vi "Init_Adapter_TCP.vi"(8 "error in (no error)":errorcluster, 11 "Siemens Ctr in":T1) -> (0 "error out":errorcluster, 3 "Siemens Ctr out":T1)   [LabVIEW 2014, in "Simatic S7.lvlib"]
uses:
  Simatic S7.lvlib
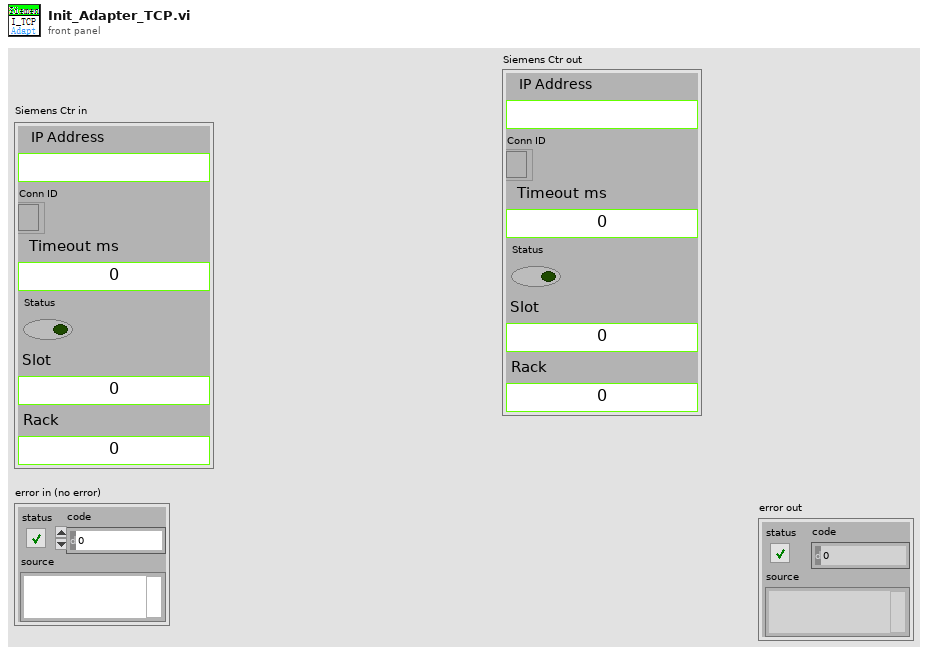
[diagram p1: front panel]
types:
  T1 = typedef "Simatic S7.lvlib/Siemens Ref.ctl" = cluster{"IP Address ":string, "Conn ID":refnum<k5>, "Timeout ms":i32, "Status":bool, "Slot":u16, "Rack":u16}
  T2 = enum16{"Standard", "Buffered", "CRLF", "Immediate"}
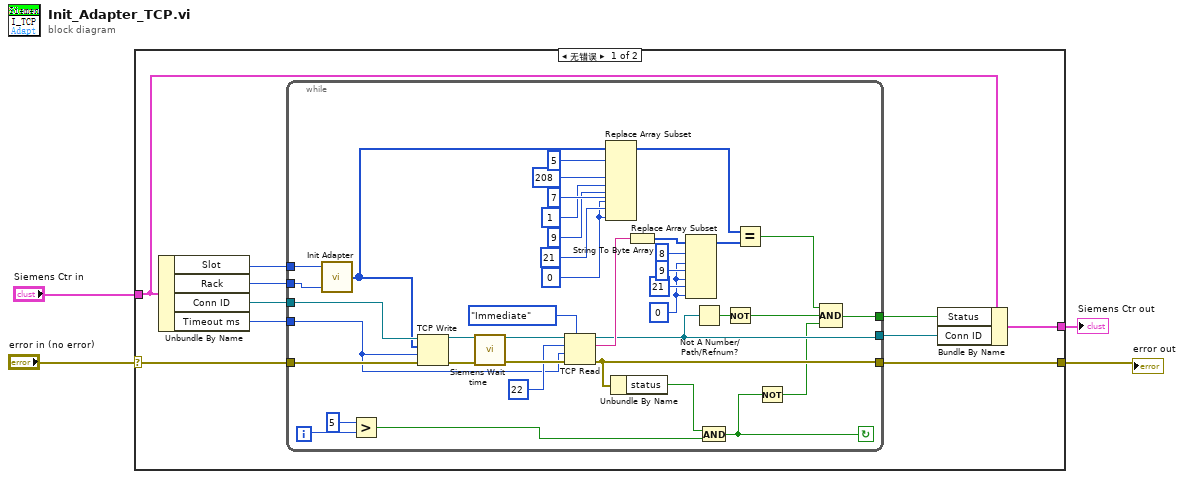
[diagram p0: block diagram]
diagram:
  n1 = case shown="无错误" "error in (no error)" {
    selector: "error in (no error)" -> [w14 w54]
    tunnel: "Siemens Ctr in" -> [w8 w53]
    tunnel: [w9 w54] -> w2
    tunnel: [w5 w53] -> w1
    frame No Error {
      n2 = Unbundle By Name(w8) -> ("Slot"=w13:u16, "Rack"=w12:u16, "Conn ID"=w11:refnum<k5>, "Timeout ms"=w10:i32)
      n3 = while {
        tunnel: w14 -> [w50]
        tunnel: w13 -> [w52]
        tunnel: w12 -> [w51]
        tunnel: w11 -> [w49]
        tunnel: w10 -> [w44]
        tunnel: [w24] -> w9
        tunnel: [w23] -> w7
        tunnel: [w15] -> w6
        i -> [w28]
        stop <- w17 continue-if-true
        w31 = u8 0 ("new element/subarray")
        w36 = u8 0 ("新元素/子数组")
        n4 = call "Init Adapter.vi"("Rack"=w51, "Slot"=w52) -> ("ISO_CR"=w35:u8[])  [unwired: 3 in]
        n5 = Greater?(x=5, y=w28) -> (0:w25:bool)
        n6 = TCP Write(connection ID=w49, data in=w35, error in (no error)=w50, 9:w44) -> (connection ID out=w46:refnum<k5>, error out=w48:errorcluster)  [unwired: 1 out]
        n7 = call "Siemens Wait time.vi"("error in (no error)"=w48) -> ("error out"=w47:errorcluster)  [unwired: 9 in, 1 out]
        n8 = TCP Read(connection ID=w46, bytes to read=22, error in (no error)=w47, 7:T2."Immediate" ("mode (standard)"), 9:w44) -> (connection ID out=w23:refnum<k5>, data out=w30:string, error out=w24:errorcluster)
        n9 = Replace Array Subset(array=w35, new element #1=u8 208 ("新元素/子数组"), index #1=5 ("索引"), new element #2=u8 1 ("新元素/子数组"), index #2=7 ("索引"), new element #3=w36, index #3=9 ("索引"), new element #4=w36, index #4=21 ("索引")) -> (w20:u8[])
        n10 = Unbundle By Name(w24) -> ("status"=w26:bool)
        n11 = String To Byte Array(string=w30) -> (unsigned byte array=w29:u8[])
        n12 = Replace Array Subset(array=w29, new element #1=w31, index #1=8 ("index"), new element #2=w31, index #2=9 ("index"), new element #3=w31, index #3=21 ("index")) -> (w21:u8[])
        n13 = Not A Number/Path/Refnum?(number/path/refnum=w23) -> (NaN/Path/Refnum?=w22:bool)
        n14 = And(x=w26, y=w25) -> (x .and. y?=w17:bool)
        n15 = Not(x=w22) -> (.not. x?=w18:bool)
        n16 = Equal?(x=w20, y=w21) -> (x = y?=w19:bool)
        n17 = Not(x=w17) -> (.not. x?=w16:bool)
        n18 = Compound Arithmetic op=AND(w19, w18, w16) -> (w15:bool)
      }
      n19 = Bundle By Name(cluster=w8, "Status"=w6, "Conn ID"=w7) -> (w5:T1)
    }
    frame Error {
    }
  }
  "error out" <- w2
  "Siemens Ctr out" <- w1
